vi "Apply Language to Project.vi"(8 "error in (no error)":errorcluster, 11 "Apply Language Wizard in":refnum<class "Apply Language Wizard.lvclass">) -> (0 "error out":errorcluster, 3 "Apply Language Wizard out":refnum<class "Apply Language Wizard.lvclass">)   [LabVIEW 2013, in "SET Project Editor.lvlib" / "Apply Language Wizard.lvclass"]
uses:
  Apply Language Wizard.lvclass
  Apply Language Wizard.lvclass/Apply Language Wizard.ctl
  UI Wizard/UI Wizard.lvclass/UI Wizard.ctl
  SET Project Data/Project Data Class/Project Data.lvclass
  SET Project Data/Resource Data Class/Resource Data.lvclass/Resource Data.ctl
  SET Project Data/VI Class/VI Data.lvclass
  SET Project Data/Resource Data Class/Read Lang LUT.vi
  UI Wizard/Read Project Data ref.vi
  SET Project Data/Resource Data Class/Resource Data.lvclass
  Lib/Printf/Messages/General/LV_Printf Msg.lvclass
  SET Project Data/Menu Class/Menu Data.lvclass
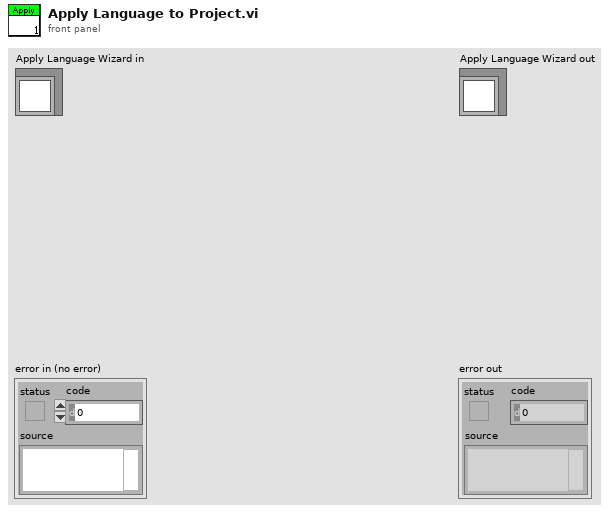
[diagram p1: front panel]
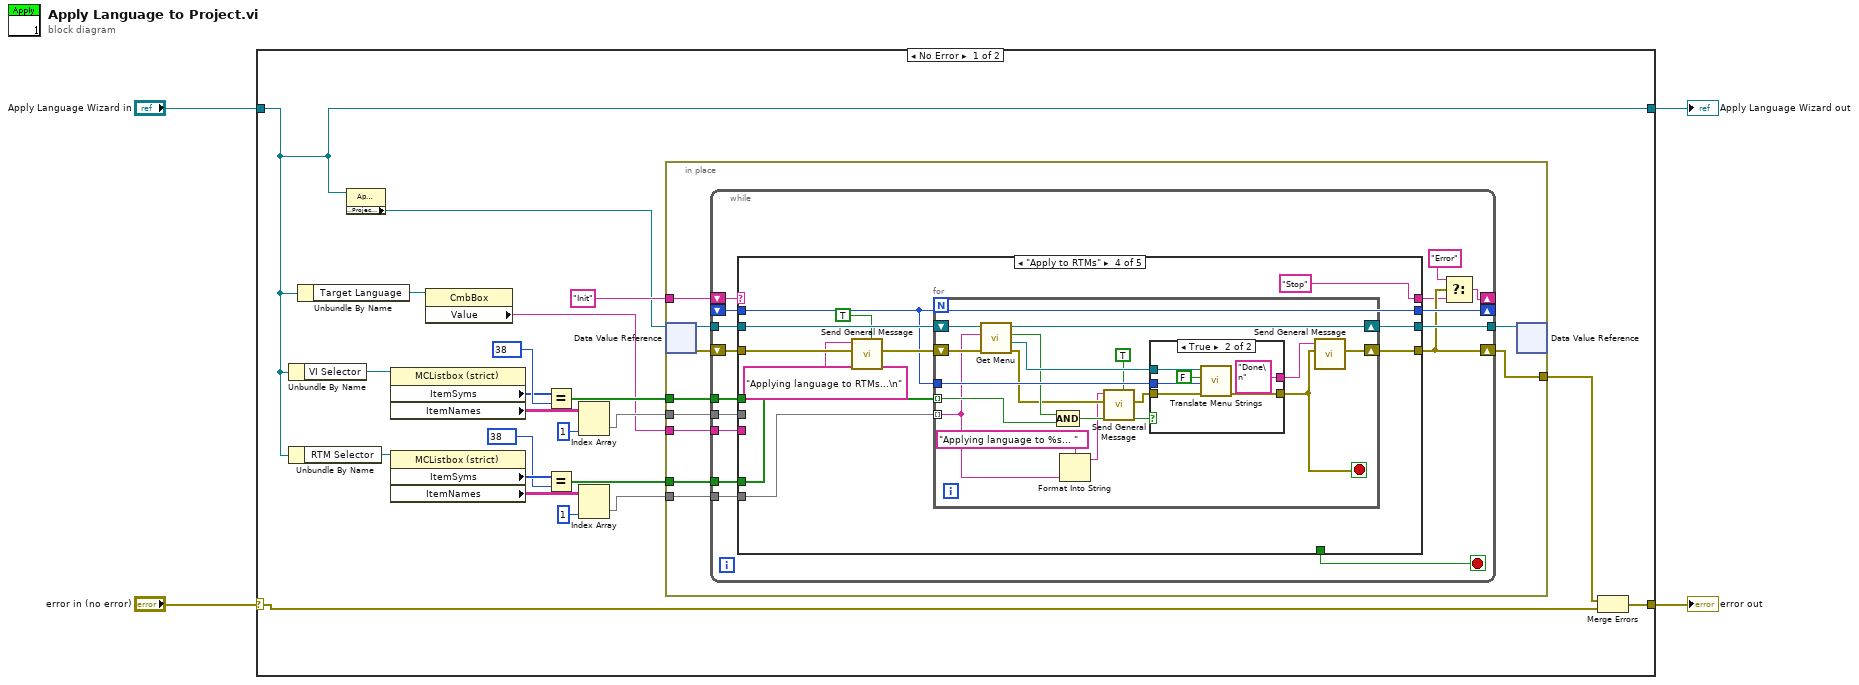
[diagram p0: block diagram]
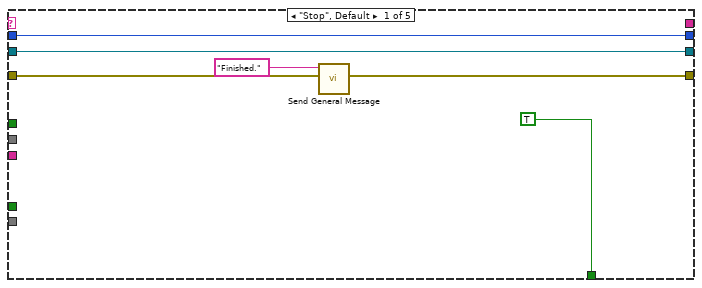
[diagram p2: hidden frame]
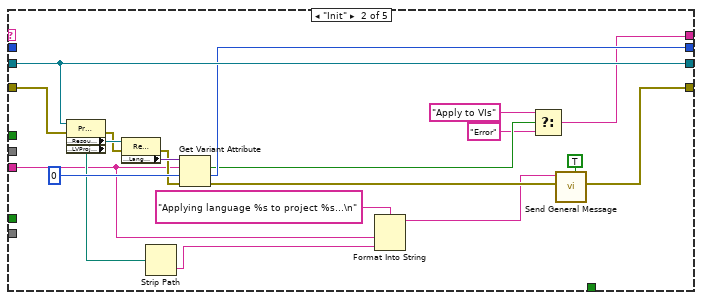
[diagram p3: hidden frame]
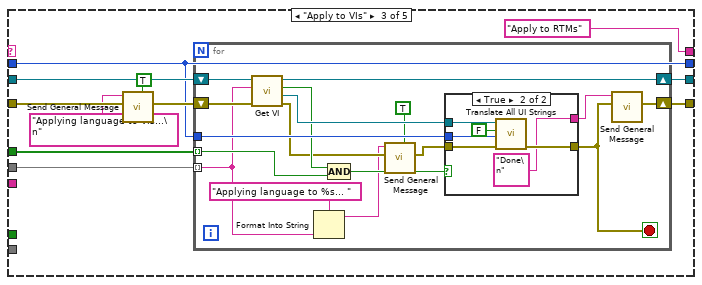
[diagram p4: hidden frame]
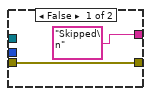
[diagram p5: hidden frame]
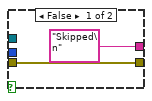
[diagram p6: hidden frame]
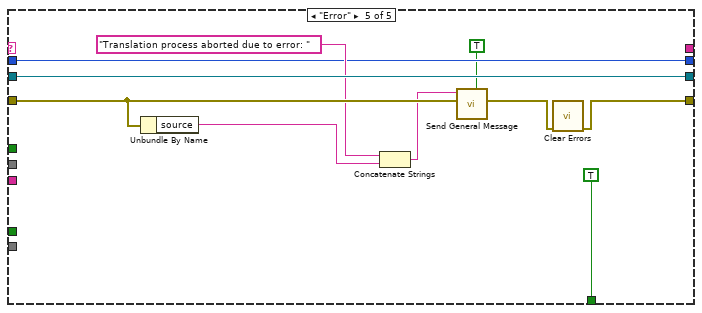
[diagram p7: hidden frame]
diagram:
  n1 = case shown="No Error" "error in (no error)" {
    selector: "error in (no error)" -> [w5 w162]
    tunnel: [w6 w162] -> w3
    tunnel: [w9 w161] -> w1
    tunnel: "Apply Language Wizard in" -> [w9 w161]
    frame No Error {
      n2 = Unbundle By Name(w9) -> ("VI Selector"=w12:refnum<vi>)
      n3 = Unbundle By Name(w9) -> ("RTM Selector"=w17:refnum<vi>)
      n4 = Unbundle By Name(w9) -> ("Target Language"=w26:refnum<vi>)
      n5 = property class="Apply Language Wizard.lvclass"(reference=w9) -> ("Properties:Project Data ref"=w8:refnum<data-value>)  [unwired: 1 in, 2 out]
      n6 = property class="MCListbox (strict)"(reference=w12) -> ("ItemSyms"=w13:i32[], "ItemNames"=w20:string[][])  [unwired: 1 in, 2 out]
      n7 = property class="MCListbox (strict)"(reference=w17) -> ("ItemSyms"=w16:i32[], "ItemNames"=w24:string[][])  [unwired: 1 in, 2 out]
      n8 = property class="CmbBox"(reference=w26) -> ("Value"=w10:string)  [unwired: 1 in, 2 out]
      n9 = Equal?(x=w13, y=38) -> (x = y?=w18:bool[])
      n10 = Equal?(x=w16, y=38) -> (x = y?=w19:bool[])
      n11 = Index Array(array=w20, index (col)=1 ("disabled index (col)")) -> (element=w22:string[])  [unwired: 1 in]
      n12 = Index Array(array=w24, index (col)=1 ("disabled index (col)")) -> (element=w25:string[])  [unwired: 1 in]
      n13 = in-place {
        in-place-border: w10 -> [w34]
        in-place-border: "Init" -> [w32]
        in-place-border: w18 -> [w31]
        in-place-border: w19 -> [w30]
        in-place-border: w22 -> [w29]
        in-place-border: [w28] -> w7
        in-place-border: w25 -> [w27]
        n14 = in-place-dvr #1(w8) -> (w35:refnum<class "Project Data.lvclass">, w33:errorcluster)
        n15 = while {
          tunnel: [w52] -> w36
          tunnel: w35 -> [w51]
          tunnel: w34 -> [w50]
          shift-right: [w38] -> _
          shift-left: w32 -> [w48]
          shift-right: [w47] -> _
          shift-left: _ -> [w46]
          shift-right: [w40] -> w28
          shift-left: w33 -> [w49]
          tunnel: w31 -> [w45]
          tunnel: w30 -> [w44]
          tunnel: w29 -> [w43]
          tunnel: w27 -> [w41]
          stop <- w42 stop-if-true
          n16 = case shown="\"Apply to RTMs\"" w48 {
            tunnel: [w58 w72 w86 w124 w160] -> w52
            tunnel: w51 -> [w58 w72 w89 w125 w160]
            tunnel: w50 -> [_ w63 _ _ _]
            tunnel: w49 -> [w55 w75 w85 w123 w158]
            tunnel: [_ w68 "Apply to RTMs" ("t") "Stop" ("t") _] -> w37
            tunnel: [w56 w71 w82 w120 w152] -> w47
            tunnel: w46 -> [w56 _ w82 w120 w152]
            tunnel: [w54 w66 w81 w119 w153] -> w40
            tunnel: w45 -> [_ _ w87 _ _]
            tunnel: w44 -> [_ _ _ w118 _]
            tunnel: w43 -> [_ _ w88 _ _]
            tunnel: [TRUE _ _ _ TRUE] -> w42
            tunnel: w41 -> [_ _ _ w117 _]
            frame "Stop", Default {
              n17 = call "Send General Message.vi"("error in (no error)"=w55, "Message"="Finished.") -> ("error out"=w54:errorcluster)  [unwired: 9 in]
            }
            frame "Init" {
              n18 = property class="Project Data.lvclass"(reference=w72, error in=w75) -> (error out=w74:errorcluster, "Properties:Resource Data ref"=w78:refnum<data-value>, "Properties:LVProject File Path"=w65:path)  [unwired: 1 out]
              n19 = property class="Resource Data.lvclass"(reference=w78, error in=w74) -> (error out=w73:errorcluster, "Properties:Lang LUT"=w77:variant)  [unwired: 1 out]
              n20 = Strip Path(path=w65) -> (name=w62:string)  [unwired: 1 out]
              n21 = Get Variant Attribute(Variant=w77, name=w63, default value (empty Variant)=0, error in=w73) -> (found=w69:bool, value=w71:i32, error out=w67:errorcluster)  [unwired: 1 out]
              n22 = Format Into String(format string="Applying language %s to project %s...\n" ("Message"), w63, w62) -> (resulting string=w61:string)  [unwired: 2 in, 1 out]
              n23 = Select(t="Apply to VIs", s=w69, f="Error") -> (s? t:f=w68:string)
              n24 = call "Send General Message.vi"("Timestamp in message? (F)"=TRUE, "error in (no error)"=w67, "Message"=w61) -> ("error out"=w66:errorcluster)  [unwired: 8 in]
            }
            frame "Apply to VIs" {
              n25 = call "Send General Message.vi"("Timestamp in message? (F)"=TRUE, "error in (no error)"=w85, "Message"="Applying language to VIs...\n") -> ("error out"=w84:errorcluster)  [unwired: 8 in]
              n26 = for {
                tunnel: w82 -> [w106]
                shift-right: [w98] -> w81
                shift-left: w84 -> [w104]
                tunnel: w88 -> [w92] mode=indexing
                tunnel: w87 -> [w100] mode=indexing
                shift-right: [w103] -> w86
                shift-left: w89 -> [w105]
                stop <- w97 stop-if-true
                n27 = call-dynamic "Get VI.vi"("error in (no error)"=w104, "VI Path (Relative)"=w92, "ProjectData in"=w105) -> ("error out"=w95:errorcluster, "VI Data out"=w102:refnum<class "VI Data.lvclass">, "found"=w101:bool, "ProjectData out"=w103:refnum<class "Project Data.lvclass">)  [unwired: 5 in]
                n28 = Format Into String(format string="Applying language to %s... " ("t"), w92) -> (resulting string=w91:string)  [unwired: 2 in, 1 out]
                n29 = Compound Arithmetic op=AND(w101, w100) -> (w99:bool)
                n30 = call "Send General Message.vi"("Timestamp in message? (F)"=TRUE, "error in (no error)"=w95, "Message"=w91) -> ("error out"=w94:errorcluster)  [unwired: 8 in]
                n31 = case shown="True" w99 {
                  tunnel: w106 -> [_ w114]
                  tunnel: w94 -> [w108 w112]
                  tunnel: [w108 w111] -> w97
                  tunnel: w102 -> [_ w110]
                  tunnel: ["Skipped\n" "Done\n"] -> w96
                  frame False {
                  }
                  frame True {
                    n32 = call-dynamic "Translate All UI Strings.vi"("error in (no error)"=w112, "Language Index (0)"=w114, "Preview?"=FALSE, "LanguageData in"=w110) -> ("error out"=w111:errorcluster)  [unwired: 6 in, 1 out]
                  }
                }
                n33 = call "Send General Message.vi"("error in (no error)"=w97, "Message"=w96) -> ("error out"=w98:errorcluster)  [unwired: 9 in]
              }
            }
            frame "Apply to RTMs" {
              n34 = call "Send General Message.vi"("Timestamp in message? (F)"=TRUE, "error in (no error)"=w123, "Message"="Applying language to RTMs...\n") -> ("error out"=w122:errorcluster)  [unwired: 8 in]
              n35 = for {
                tunnel: w120 -> [w142]
                shift-right: [w134] -> w119
                shift-left: w122 -> [w140]
                tunnel: w117 -> [w128] mode=indexing
                tunnel: w118 -> [w136] mode=indexing
                shift-right: [w139] -> w124
                shift-left: w125 -> [w141]
                stop <- w133 stop-if-true
                n36 = call-dynamic "Get Menu.vi"("error in (no error)"=w140, "Menu Path (Relative)"=w128, "ProjectData in"=w141) -> ("error out"=w131:errorcluster, "Menu Data out"=w138:refnum<class "Menu Data.lvclass">, "found"=w137:bool, "ProjectData out"=w139:refnum<class "Project Data.lvclass">)  [unwired: 5 in]
                n37 = Compound Arithmetic op=AND(w137, w136) -> (w135:bool)
                n38 = Format Into String(format string="Applying language to %s... ", w128) -> (resulting string=w127:string)  [unwired: 2 in, 1 out]
                n39 = call "Send General Message.vi"("Timestamp in message? (F)"=TRUE, "error in (no error)"=w131, "Message"=w127) -> ("error out"=w130:errorcluster)  [unwired: 8 in]
                n40 = case shown="True" w135 {
                  tunnel: w142 -> [_ w150]
                  tunnel: w130 -> [w144 w148]
                  tunnel: [w144 w147] -> w133
                  tunnel: w138 -> [_ w146]
                  tunnel: ["Skipped\n" "Done\n"] -> w132
                  frame False {
                  }
                  frame True {
                    n41 = call "Translate Menu Strings.vi"("error in (no error)"=w148, "Language Index (0)"=w150, "Preview?"=FALSE, "Menu Data in"=w146) -> ("error out"=w147:errorcluster)  [unwired: 5 in, 2 out]
                  }
                }
                n42 = call "Send General Message.vi"("error in (no error)"=w133, "Message"=w132) -> ("error out"=w134:errorcluster)  [unwired: 9 in]
              }
            }
            frame "Error" {
              n43 = Unbundle By Name(w158) -> ("source"=w156:string)
              n44 = Concatenate Strings("Translation process aborted due to error: " ("Message"), w156) -> (w155:string)
              n45 = call "Send General Message.vi"("Timestamp in message? (F)"=TRUE, "error in (no error)"=w158, "Message"=w155) -> ("error out"=w154:errorcluster)  [unwired: 8 in]
              n46 = call <vilib>:"Clear Errors.vi"("error in (no error)"=w154) -> ("error out"=w153:errorcluster)  [unwired: 6 in]
            }
          }
          n47 = Select(t="Error", s=w40, f=w37) -> (s? t:f=w38:string)
        }
        n48 = in-place-dvr #1(w36) -> ()  [unwired: 2 out]
      }
      n49 = Merge Errors(w7, w5) -> (w6:errorcluster)
    }
    frame Error {
    }
  }
  "error out" <- w3
  "Apply Language Wizard out" <- w1
